vi "历史数据回显.vi"() -> ()   [LabVIEW 2012]
uses:
  <vilib>/Utility/file.llb/Read From Spreadsheet File (DBL).vi
panel:
  out "转速波形":dbl[](graph)
  out "电流波形":dbl[](graph)
  out "电压波形":dbl[](graph)
  in  "数据存储路径":path=path "E:/数据保存"
  in  "显示":bool
  in  "返回":bool
  # "历史数据显示"
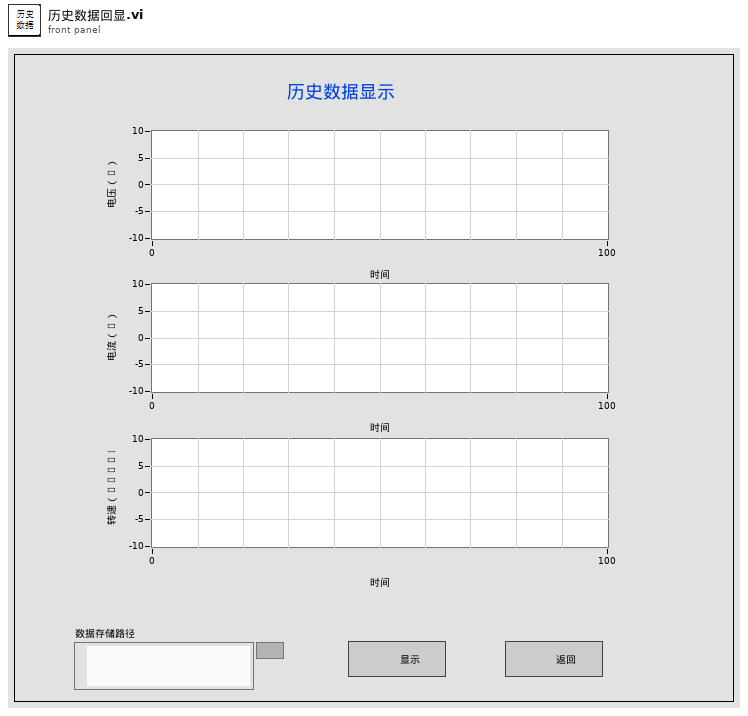
[diagram p1: front panel]
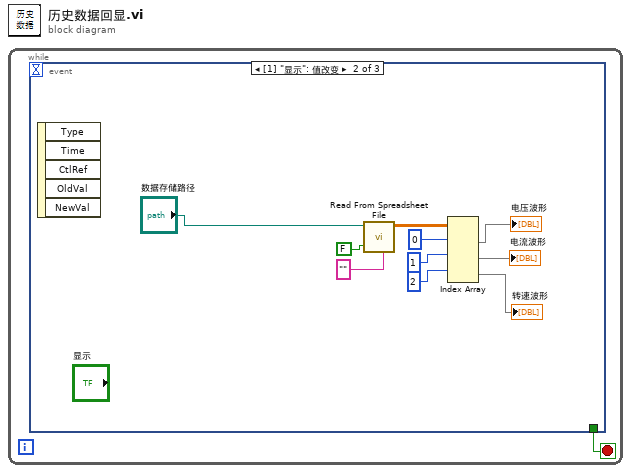
[diagram p0: block diagram]
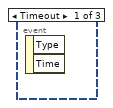
[diagram p2: hidden frame]
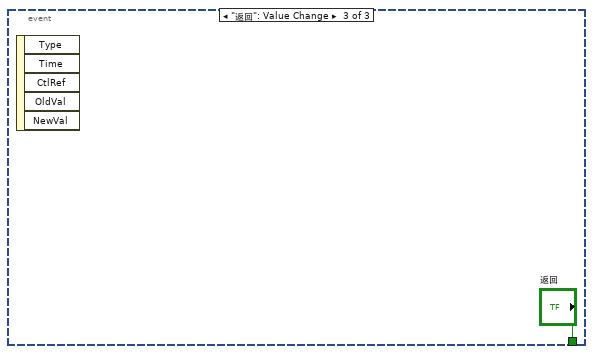
[diagram p3: hidden frame]
diagram:
  n1 = while {
    stop <- w1 stop-if-true
    n2 = event shown="[1] \"显示\": 值改变" {
      selector: _ -> [_ _ _]
      dyn-events: _ -> [_ _ _]
      timeout: _ -> [_ _ _]
      tunnel: [_ _ "返回"] -> w1
      event Timeout {
        n3 = event-data() -> ()  [unwired: 1 in, 2 out]
      }
      event "显示": Value Change {
        n4 = event-data() -> ()  [unwired: 1 in, 5 out]
        n5 = call-poly <vilib>:"Read From Spreadsheet File.vi"("delimiter (\\t)"="" ("delimiter (\\t)"), "transpose (no:F)"=FALSE ("append to file? (new file:F)"), "file path (dialog if empty)"="数据存储路径") -> ("all rows"=w8:dbl[][])  [unwired: 4 in, 4 out]
        n6 = Index Array(array=w8, index (row) #1=0 ("禁用的索引 (列)"), index (row) #2=1 ("禁用的索引 (列)"), index (row) #3=2 ("禁用的索引 (列)")) -> (element #1=→"电压波形":dbl[], element #2=→"电流波形":dbl[], element #3=→"转速波形":dbl[])  [unwired: 3 in]
      }
      event "返回": Value Change {
        n7 = event-data() -> ()  [unwired: 1 in, 5 out]
      }
    }
  }
